vi "Show All Hardware_MOD.vi"() -> ()   [LabVIEW 2021]
doc: "Displays all hardware and certain properties of that hardware on the specified target."
uses:
  <vilib>/Utility/error.llb/DialogType.ctl
  <vilib>/nisyscfg/Filter Mode.ctl
  786f16a0-9eb0-424a-b110-95e7cb814a15.vi
  <vilib>/Array/Sort 2D Array - Pop Stack.vi
  <vilib>/Array/Sort 2D Array - Push Stack.vi
  <vilib>/nisyscfg/Close (Hardware).vi
  <vilib>/nisyscfg/Close (Filter).vi
  <vilib>/nisyscfg/Close (System).vi
  <vilib>/nisyscfg/nisyscfg.lvlib
  <resource>/objmgr/niflexrioatomicsae.rc
  <resource>/objmgr/nicontrollersysapi.rc
  <instrlib>/niScope/Utility/niScope Get Channel Name.vi
panel:
  out "LoopCount":i32
  out "Array 2":string[](array[string])
  in  "User Name":string
  in  "Password":string
  in  "Target (localhost)":refnum<k21>="localhost"
  in  "Show All Network Devices":bool
  out "Resources":string[][](table)
  # "Overview: Displays all hardware and certain properties of that hardware on the specified target.\nRequirements: NI System Configuration, applicable device drivers\nInstructions:\n1. Select Target. Enter User Name and Password if necessary.\n2. Run the VI."
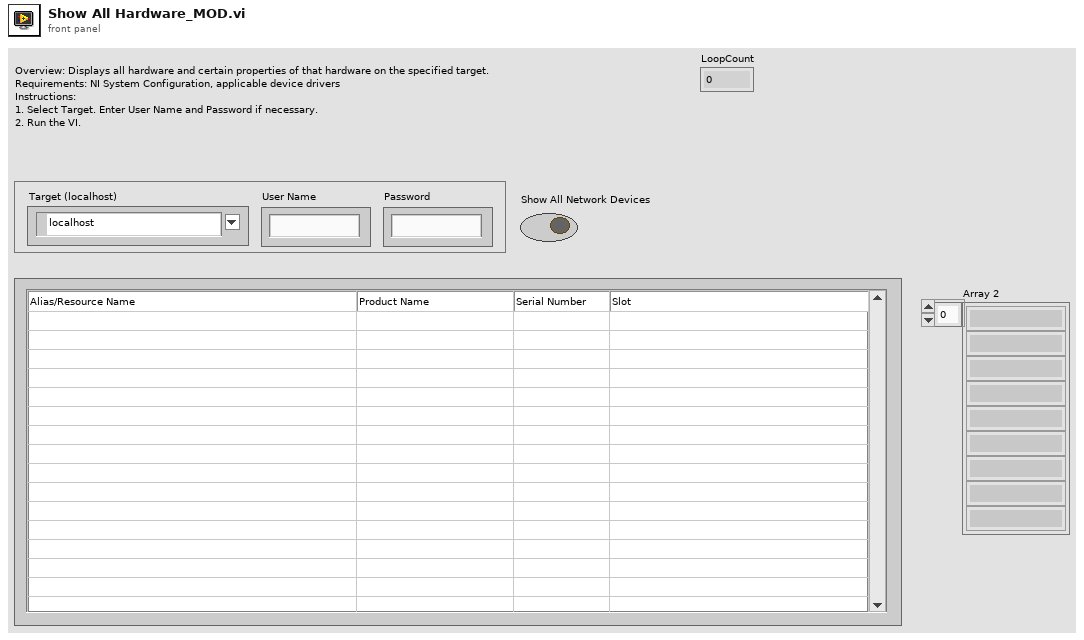
[diagram p1: front panel]
types:
  T1 = typedef "nisyscfg.lvlib/Filter Mode.ctl" = i32
  T2 = typedef "DialogType.ctl" = u16
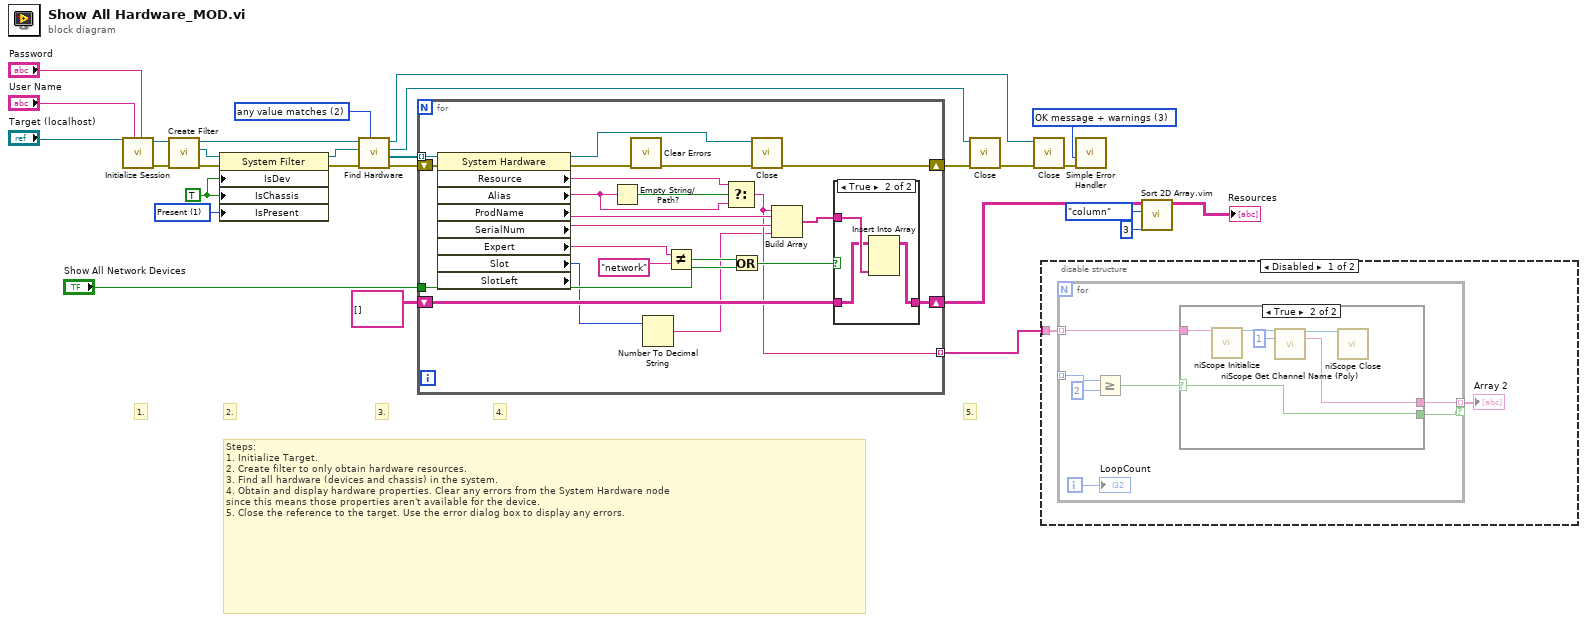
[diagram p0: block diagram]
diagram:
  w6 = 1 items=["Initializing"=-2, "Unknown"=-1, "Not Present"=0, "Present"=1] ("Devices & Chassis:Is Present")
  w15 = T1 2 items=["all values match"=1, "any value matches"=2, "values do not match"=3, "all properties exist"=4] ("filter mode (all values match)")
  w7 = TRUE ("Is Chassis")
  w23 = T2 3 items=["no dialog", "OK message", "continue or stop message", "OK message + warnings", "continue/stop + warnings"] ("type of dialog (OK msg:1)")
  # "2."
  # "5."
  # "4."
  # "3."
  # "1."
  # "Steps:\n1. Initialize Target.\n2. Create filter to only obtain hardware resources.\n3. Find all hardware (devices and chassis) in the system.\n4. Obtain and display hardware properties. Clear any errors from the System Hardware node\nsince this means those properties aren't available for the device. \n5. Close the reference to the target. Use the error dialog box to display any errors."
  n1 = call <vilib>:"Initialize Session.vi"("Password"="Password", "User Name"="User Name", "Target (localhost)"="Target (localhost)") -> ("error out"=w17:errorcluster, "Session out"=w20:refnum<k21>)  [unwired: 7 in]
  n2 = call <vilib>:"Create Filter.vi"("error in (no error)"=w17, "Session in"=w20) -> ("error out"=w22:errorcluster, "Filter out"=w21:refnum<k20>, "Session out"=w19:refnum<k21>)  [unwired: 7 in]
  n3 = property class="System Filter"(reference=w21, error in=w22, "IsDev"=w7, "IsChassis"=w7, "IsPresent"=w6) -> (reference out=w16:refnum<k20>, error out=w18:errorcluster)
  n4 = call <vilib>:"Find Hardware.vi"("Filter Mode (all values match)"=w15, "error in (no error)"=w18, "Filter in"=w16, "Session in"=w19) -> ("error out"=w11:errorcluster, "Resources out"=w28:refnum<k20>[], "Filter out"=w13:refnum<k20>, "Session out"=w24:refnum<k21>)  [unwired: 4 out]
  n5 = for {
    tunnel: w28 -> [w48] mode=indexing
    shift-right: [w50] -> w12
    shift-left: w11 -> [w41]
    shift-right: [w40] -> w4
    shift-left: string[][] [] ("Results") -> [w38]
    tunnel: "Show All Network Devices" -> [w33]
    tunnel: [w31] -> w5 mode=indexing
    n6 = property class="System Hardware" props=["Resource", "Alias", "ProdName", "SerialNum", "Expert", "Slot", "SlotLeft"](reference=w48, error in=w41) -> (reference out=w42:refnum<k20>, error out=w43:errorcluster, "Resource"=w46:string, "Alias"=w47:string, "ProdName"=w45:string, "SerialNum"=w44:string, "Expert"=w37:string, "Slot"=w30:i32)  [unwired: 1 out]
    n7 = Empty String/Path?(string/path=w47) -> (empty?=w49:bool)
    n8 = call <vilib>:"Clear Errors.vi"("error in (no error)"=w43) -> ("error out"=w32:errorcluster)  [unwired: 5 in, 1 out]
    n9 = Number To Decimal String(number=w30) -> (decimal integer string=w29:string)  [unwired: 1 in]
    n10 = Not Equal?(x=w37, y="network") -> (x != y?=w34:bool)
    n11 = Select(t=w46, s=w49, f=w47) -> (s? t:f=w31:string)
    n12 = Or(x=w34, y=w33) -> (x .or. y?=w35:bool)
    n13 = call-poly <vilib>:"Close.vi"("error in (no error)"=w32, "Resource in"=w42) -> ("error out"=w50:errorcluster)  [unwired: 9 in]
    n14 = Build Array(w31, w45, w44, w29) -> (w39:string[])
    n15 = case shown="True" w35 {
      tunnel: [w51 w54] -> w40
      tunnel: w39 -> [_ w53]
      tunnel: w38 -> [w51 w52]
      frame False {
      }
      frame True {
        n16 = Insert Into Array(array=w52, new element=w53) -> (w54:string[][])  [unwired: 2 in]
      }
    }
  }
  n17 = call-poly <vilib>:"Close.vi"("error in (no error)"=w12, "Filter in"=w13) -> ("error out"=w14:errorcluster)  [unwired: 9 in]
  n18 = call-poly <vilib>:"Close.vi"("error in (no error)"=w14, "Session in"=w24) -> ("error out"=w27:errorcluster)  [unwired: 9 in]
  n19 = disable-structure shown="Disabled" {
    disable-tunnel: w5 -> [w56 _]
    frame Disabled {
      n20 = for {
        tunnel: w56 -> [w63] mode=indexing
        tunnel: [w62] -> w55 mode=indexing if=w58
        tunnel: _ -> [w61] mode=indexing
        i -> [w57]
        n21 = Greater Or Equal?(x=w61, y=2) -> (x >= y?=w59:bool)
        n22 = case shown="True" w59 {
          selector: w59 -> [w64 w65]
          tunnel: w63 -> [_ w70]
          tunnel: [_ w67] -> w62
          tunnel: [w64 w65] -> w58
          frame False {
          }
          frame True {
            n23 = call <instrlib>:"niScope Initialize.vi"("resource name"=w70) -> ("instrument handle"=w69:refnum<k15>)  [unwired: 13 in, 1 out]
            n24 = call-poly <instrlib>:"niScope Get Channel Name (Poly).vi"("instrument handle"=w69, "index"=1) -> ("instrument handle out"=w68:refnum<k15>, "channel name"=w67:string)  [unwired: 11 in, 1 out]
            n25 = call <instrlib>:"niScope Close.vi"("instrument handle"=w68) -> ()  [unwired: 14 in, 1 out]
          }
        }
        "LoopCount" <- w57
      }
      "Array 2" <- w55
    }
    frame Enabled {
    }
  }
  n26 = call <vilib>:"Simple Error Handler.vi"("type of dialog (OK msg:1)"=w23, "error in (no error)"=w27) -> ()  [unwired: 3 in, 5 out]
  n27 = call "Sort 2D Array.vim"("index"=3, "dimension to index (column)"=enum16{"column", "row"}."column", "2D array"=w4) -> ("sorted 2D array"=→"Resources":string[][])  [unwired: 7 in, 1 out]
